vi "writeString.vi"(8 "error in (no error)":errorcluster, 10 "Input":string, 11 "M1M3SAL in":refnum<class "M1M3SAL.lvclass">) -> (0 "error out":errorcluster, 3 "M1M3SAL out":refnum<class "M1M3SAL.lvclass">)   [LabVIEW 2016, in "M1M3SupportCommunicator.lvlib" / "M1M3SAL.lvclass"]
uses:
  M1M3SAL.lvclass
  M1M3SAL.lvclass/M1M3SAL.ctl
  writeU8.vi
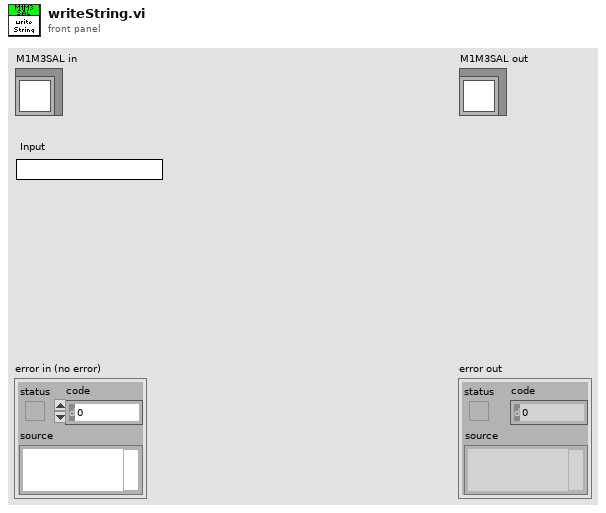
[diagram p1: front panel]
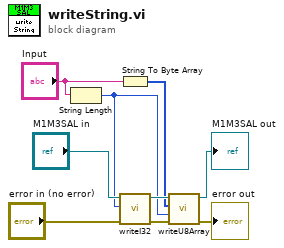
[diagram p0: block diagram]
diagram:
  n1 = String Length(string="Input") -> (length=w5:i32)
  n2 = String To Byte Array(string="Input") -> (unsigned byte array=w6:u8[])
  n3 = call "writeI32.vi"("error in (no error)"="error in (no error)", "Input"=w5, "M1M3SAL in"="M1M3SAL in") -> ("error out"=w2:errorcluster, "M1M3SAL out"=w7:refnum<class "M1M3SAL.lvclass">)  [unwired: 7 in]
  n4 = call "writeU8Array.vi"("error in (no error)"=w2, "Length"=w5, "Input"=w6, "M1M3SAL in"=w7) -> ("error out"=→"error out":errorcluster, "M1M3SAL out"=→"M1M3SAL out":refnum<class "M1M3SAL.lvclass">)  [unwired: 6 in]
